vi "Benchmark SV Send  LV2012 - NI Verified - 100 Byte - 1Var.vi"() -> ()   [LabVIEW 2015]
uses:
  <vilib>/Platform/TimedLoop/XDataNode/timing_clust.ctl
  <vilib>/Platform/TimedLoop/XDataNode/nitl_modes.ctl
  <vilib>/Platform/TimedLoop/XDataNode/wakeup.ctl
  <vilib>/platform/TimedLoop/XDataNode/XDataNode.xnode
  <vilib>/Platform/TimedLoop/XDataNode/XDNodeRunTimeDep.lvlib
panel:
  out "100 byte":i32[][](array[numeric])
  out "Time":u32
  in  "stop 2":bool
  out "Delay (ms)":u32
  out "Average Delay (ms)":dbl
  out "Tries":u32
  # "Overview:  Coding that exemplifies how to benchmark the communication of Shared Variables.\nRequirements: LabVIEW 2012 or compatible\nInstructions:\n1.  Run the \"Benchmark SV Receive LV2012 - NI Verified.vi\"\n2. Run this VI\n3. Watch the amount of time it takes to communicate\n4. Stop both VIs"
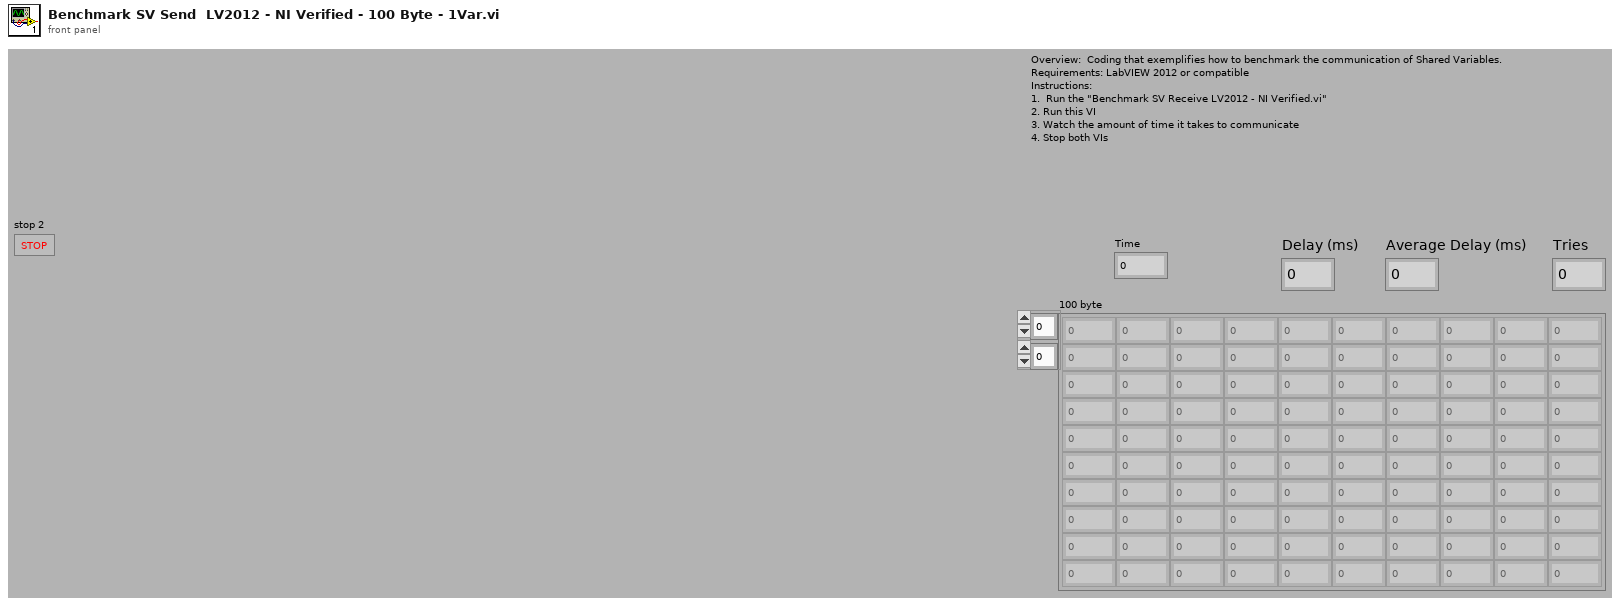
[diagram p1: front panel]
types:
  T1 = typedef "XDNodeRunTimeDep.lvlib/timing_clust.ctl" = cluster{"Expected End [f-1]":u64, "Actual End [f-1]":u64, "Finished Late? [f-1]":bool, "Expected End [i-1]":u64, "Actual End [i-1]":u64, "Finished Late? [i-1]":bool, "Expected Start [i]":u64, "Actual Start [i]":u64, "Expected Start [f]":u64, "Actual Start [f]":u64, "Source Name":string, "Structure Name":string, "Period":i64, "Deadline":i64, "Offset":i64, "Start":i64, "Priority":i32, "Timeout":i32, "Mode":T2, "Wakeup Reason":T3, "Error":errorcluster, "Source Type":string, "Secondary Source Type":string, "Global End Time":u64, "Global Start Time":u64, "Frame Duration":u64, "Iteration Duration":u64, "Assigned CPU":i32, "I/O Scan Engine Mode":u32}
  T2 = typedef "XDNodeRunTimeDep.lvlib/nitl_modes.ctl" = enum32{"No Change", "Process missed periods, maintain original phase", "Discard missed periods, maintain original phase", "Process missed periods, ignore original phase", "Discard missed periods, ignore original phase"}
  T3 = typedef "XDNodeRunTimeDep.lvlib/wakeup.ctl" = enum32{"Normal", "Aborted", "Asynchronous wakeup", "Timing source error", "Timed loop error", "Timeout"}
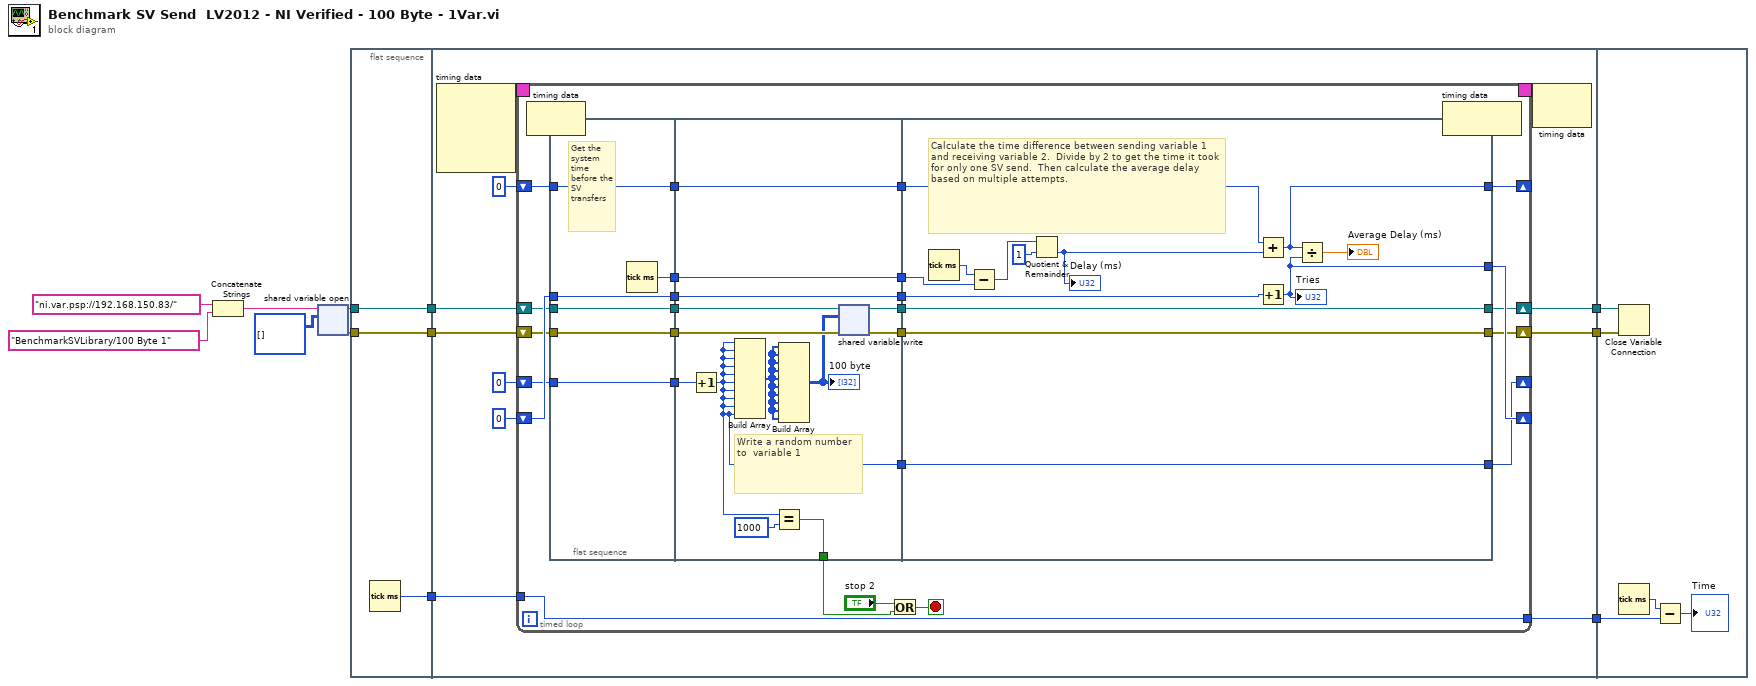
[diagram p0: block diagram]
diagram:
  n1 = Concatenate Strings("ni.var.psp://192.168.150.83/" ("string"), "BenchmarkSVLibrary/100 Byte 1") -> (w6:string)
  n2 = shared-variable-open(w6, i32[][] [] ("appended array")) -> (w4:refnum<k21>, w5:errorcluster)  [unwired: 2 in]
  n3 = flat-sequence {
    tunnel: w4 -> [w14]
    tunnel: w5 -> [w15]
    tunnel: [w15] -> w12
    tunnel: [w14] -> w11
    tunnel: [w13] -> w10
    tunnel: [w21] -> w9
    tunnel: w12 -> [w23]
    tunnel: w11 -> [w22]
    tunnel: w10 -> [w20]
    tunnel: [w19] -> w8
    tunnel: [w18] -> w7
    tunnel: w9 -> [w91]
    tunnel: w8 -> [w90]
    tunnel: w7 -> [w89]
    frame #0 {
      n4 = Tick Count (ms)() -> (millisecond timer value=w13:u32)
    }
    frame #1 {
      n5 = node-c288() -> (w17:T1)  [unwired: 4 in]
      n6 = timed-loop {
        shift-right: [w52] -> _
        shift-left: u32 0 -> [w46]
        shift-right: [w51] -> _
        shift-left: u32 0 -> [w47]
        shift-right: [w43] -> _
        shift-left: u64 0 -> [w44]
        shift-right: [w35] -> w19
        shift-left: w23 -> [w33]
        shift-right: [w30] -> w18
        shift-left: w22 -> [w28]
        tunnel: [w27] -> w21
        tunnel: w20 -> [w27]
        timing: w17 -> [_]
        timing-out: [_] -> w16
        stop <- w42 stop-if-true
        n7 = node-c288() -> ()  [unwired: 1 in, 1 out]
        n8 = flat-sequence {
          tunnel: [w58] -> w50
          tunnel: [w60] -> w49
          tunnel: [w59] -> w48
          tunnel: [w57] -> w45
          tunnel: [w56] -> w32
          tunnel: [w55] -> w31
          tunnel: w46 -> [w60]
          tunnel: w47 -> [w59]
          tunnel: w44 -> [w57]
          tunnel: w33 -> [w56]
          tunnel: w28 -> [w55]
          tunnel: [w73] -> w39
          tunnel: [w72] -> w38
          tunnel: [w71] -> w37
          tunnel: w50 -> [w73]
          tunnel: w49 -> [w72]
          tunnel: w48 -> [w71]
          tunnel: w45 -> [w70]
          tunnel: [w62] -> w36
          tunnel: [w68] -> w40
          tunnel: [w67] -> w34
          tunnel: w32 -> [w66]
          tunnel: w31 -> [w65]
          tunnel: [w64] -> w29
          tunnel: w39 -> [w85]
          tunnel: [w78] -> w52
          tunnel: w38 -> [w80]
          tunnel: [w77] -> w51
          tunnel: w37 -> [w84]
          tunnel: w36 -> [w76]
          tunnel: [w76] -> w43
          tunnel: [w75] -> w35
          tunnel: w34 -> [w75]
          tunnel: [w74] -> w30
          tunnel: w29 -> [w74]
          frame #0 {
            # "Get the system time before the SV transfers"
            n9 = Tick Count (ms)() -> (millisecond timer value=w58:u32)
          }
          frame #1 {
            # "Write a random number to  variable 1"
            n10 = Increment(x=w70) -> (x+1=w62:u64)
            n11 = Build Array(w62, w62, w62, w62, w62, w62, w62, w62, w62, w62) -> (w63:u64[])
            n12 = Equal?(x=w62, y=u64 1000) -> (x = y?=w68:bool)
            n13 = Build Array(w63, w63, w63, w63, w63, w63, w63, w63, w63, w63) -> (w61:u64[][])
            "100 byte" <- w61
            n14 = shared-variable-write(w65, w66, w61) -> (w64:refnum<k21>, w67:errorcluster)
          }
          frame #2 {
            # "Calculate the time difference between sending variable 1 and receiving variable 2.  Divide by 2 to get the time it took for only one SV send.  Then calculate the average delay based on multiple attempts."
            n15 = Tick Count (ms)() -> (millisecond timer value=w86:u32)
            n16 = Subtract(x=w86, y=w85) -> (x-y=w83:u32)
            n17 = Quotient & Remainder(x=w83, y=u32 1) -> (floor(x/y)=w81:u32)  [unwired: 1 out]
            "Delay (ms)" <- w81
            n18 = Add(x=w80, y=w81) -> (x+y=w78:u32)
            n19 = Increment(x=w84) -> (x+1=w77:u32)
            "Tries" <- w77
            n20 = Divide(x=w78, y=w77) -> (x/y=→"Average Delay (ms)":dbl)
          }
        }
        n21 = Or(x="stop 2", y=w40) -> (x .or. y?=w42:bool)
        n22 = node-c288() -> ()  [unwired: 1 in, 1 out]
      }
      n23 = node-c288(w16) -> ()  [unwired: 1 out]
    }
    frame #2 {
      n24 = Close Variable Connection(8:w90, 11:w89) -> ()  [unwired: 1 out]
      n25 = Tick Count (ms)() -> (millisecond timer value=w93:u32)
      n26 = Subtract(x=w93, y=w91) -> (x-y=→"Time":u32)
    }
  }
